vi "Revision Query.vi"(8 "error in (no error)":errorcluster, 10 "Device Number":u8, 11 "VISA resource name":refnum<visa-resource-name>) -> (0 "error out":errorcluster, 1 "Instrument Firmware Revision":string, 2 "Instrument Driver Revision":string, 3 "VISA resource name out":refnum<visa-resource-name>)   [LabVIEW 2015, in "ZaberTSeries.lvlib"]
doc: "Queries the current instrument firmware revision and instrument driver revision.\n\nFor detailed driver information including modification history, refer to the Readme file."
uses:
  ZaberTSeries.lvlib
  Request.ctl
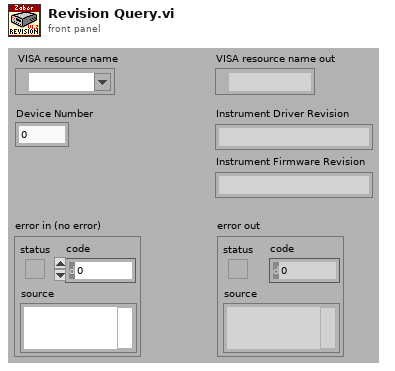
[diagram p1: front panel]
types:
  T1 = typedef "ZaberTSeries.lvlib/Request.ctl" = cluster{"Device Number":u8, "Command":u8, "Data":i32, "Response Count":i32}
  T2 = typedef "ZaberTSeries.lvlib/Response.ctl" = cluster{"Device Number":u8, "Command":u8, "Data":i32}
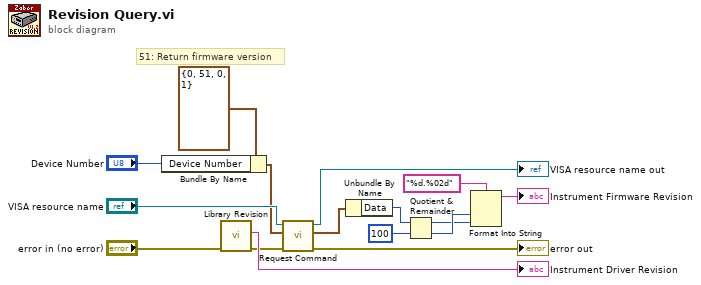
[diagram p0: block diagram]
diagram:
  # "51: Return firmware version"
  n1 = Bundle By Name(cluster=T1 {"Device Number"=0, "Command"=51, "Data"=0, "Response Count"=1} ("Request"), "Device Number"="Device Number") -> (w10:T1)
  n2 = call "Library Revision.vi"("error in (no error)"="error in (no error)") -> ("error out"=w13:errorcluster, "Library Revision"=→"Instrument Driver Revision":string)  [unwired: 9 in]
  n3 = call "Request Command.vi"("error in (no error)"=w13, "Request"=w10, "VISA resource name"="VISA resource name") -> ("error out"=→"error out":errorcluster, "First Response"=w8:T2, "VISA resource name out"=→"VISA resource name out":refnum<visa-resource-name>)  [unwired: 5 in, 1 out]
  n4 = Unbundle By Name(w8) -> ("Data"=w7:i32)
  n5 = Quotient & Remainder(x=w7, y=100) -> (x-y*floor(x/y)=w2:i32, floor(x/y)=w3:i32)
  n6 = Format Into String(format string="%d.%02d", w3, w2) -> (resulting string=→"Instrument Firmware Revision":string)  [unwired: 2 in, 1 out]
